vi "Alias Format Specifier.vi"() -> (2 "Alias Format specifier":string, 3 "Default Alias":string)   [LabVIEW 2020]
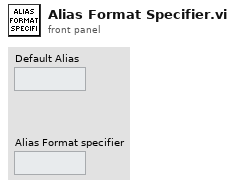
[diagram p1: front panel]
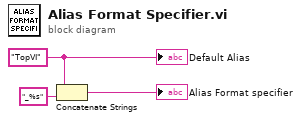
[diagram p0: block diagram]
diagram:
  w1 = "TopVI" ("Tag Name")
  n1 = Concatenate Strings(w1, "_%s" ("string")) -> (→"Alias Format specifier":string)
  "Default Alias" <- w1
